vi "Simulation.vi"() -> ()   [LabVIEW 2012]
uses:
  <vilib>/Simulation/Scripting/Companion Diagram/SimConfigNode/SimParams.ctl
  <vilib>/Simulation/Scripting/Companion Diagram/SimConfigNode/_simSolvers.ctl
  <vilib>/Simulation/Implementation/Shared/SIMSCR Execution Mode.ctl
  <vilib>/Simulation/Param Hierarchy/Typedefs/SIMPH Param Control Actions.ctl
  <vilib>/Simulation/Implementation/Shared/NILVSim_ParamChanged.vi
  <vilib>/Simulation/ContinuousLinear/Implementation/NILVSim Transfer Function.llb/SIM Transfer Function Distributor (SISO).vi
  <vilib>/Simulation/DiscreteLinear/Implementation/NILVSim Discrete ZOH.llb/SIM Discrete ZOH (scalar).vi
  <vilib>/Simulation/Nonlinear/Implementation/NILVSim Relay.llb/SIM Relay (scalar).vi
  <vilib>/Simulation/ContinuousLinear/Implementation/NILVSim Transfer Function.llb/SIM Transfer Function Collector (SISO).vi
  <vilib>/Simulation/SignalDisplay/Implementation/NILVSim Time Waveform.llb/SIM Time Waveform (scalar).vi
  <vilib>/Simulation/Implementation/Shared/NILVSim_Manager.vi
  <vilib>/Simulation/Implementation/Shared/NILVSim_FinalizeModel.vi
  <vilib>/Simulation/Implementation/Shared/SIM Unbundle Sim Info.vi
  <vilib>/Utility/error.llb/Clear Errors.vi
  <vilib>/Simulation/Implementation/Shared/NILVSim_GetModelError.vi
  <vilib>/Simulation/Implementation/Shared/SIM Bundle Sim Info.vi
  <vilib>/Simulation/Implementation/Shared/SIMSH Read Queue.vi
  <vilib>/Simulation/Implementation/Shared/NILVSim_Initialize.vi
  <vilib>/Simulation/Utility/Implementation/NILVSim Get Time and IsAcceptedStep.vi
  <vilib>/Simulation/Scripting/Companion Diagram/SimConfigNode/SimDog.xnode
  <vilib>/Simulation/Implementation/XNodeFramework/SimXNode/SimX.xnode
  <vilib>/Simulation/ContinuousLinear/Implementation/NILVSim Transfer Function.llb/SIM Transfer Function (SISO).vi
  <vilib>/Simulation/Implementation/Shared/NI_SIM_Implementation.lvlib
panel:
  in  "sample  time":dbl
  in  "Lower Limit":dbl
  in  "Upper Limit":dbl
  in  "Off Voltage":dbl
  in  "Suply Voltage":dbl
  out "Output":dbl(slide) scale=0.0..5.0
  out "Controlled Variable (Plant output)":waveform(dbl)(graph)={"t0"=timestamp(9343.2 s since 1904-01-01), "dt"=1.0, "Y"=[0.2633720690985406]}
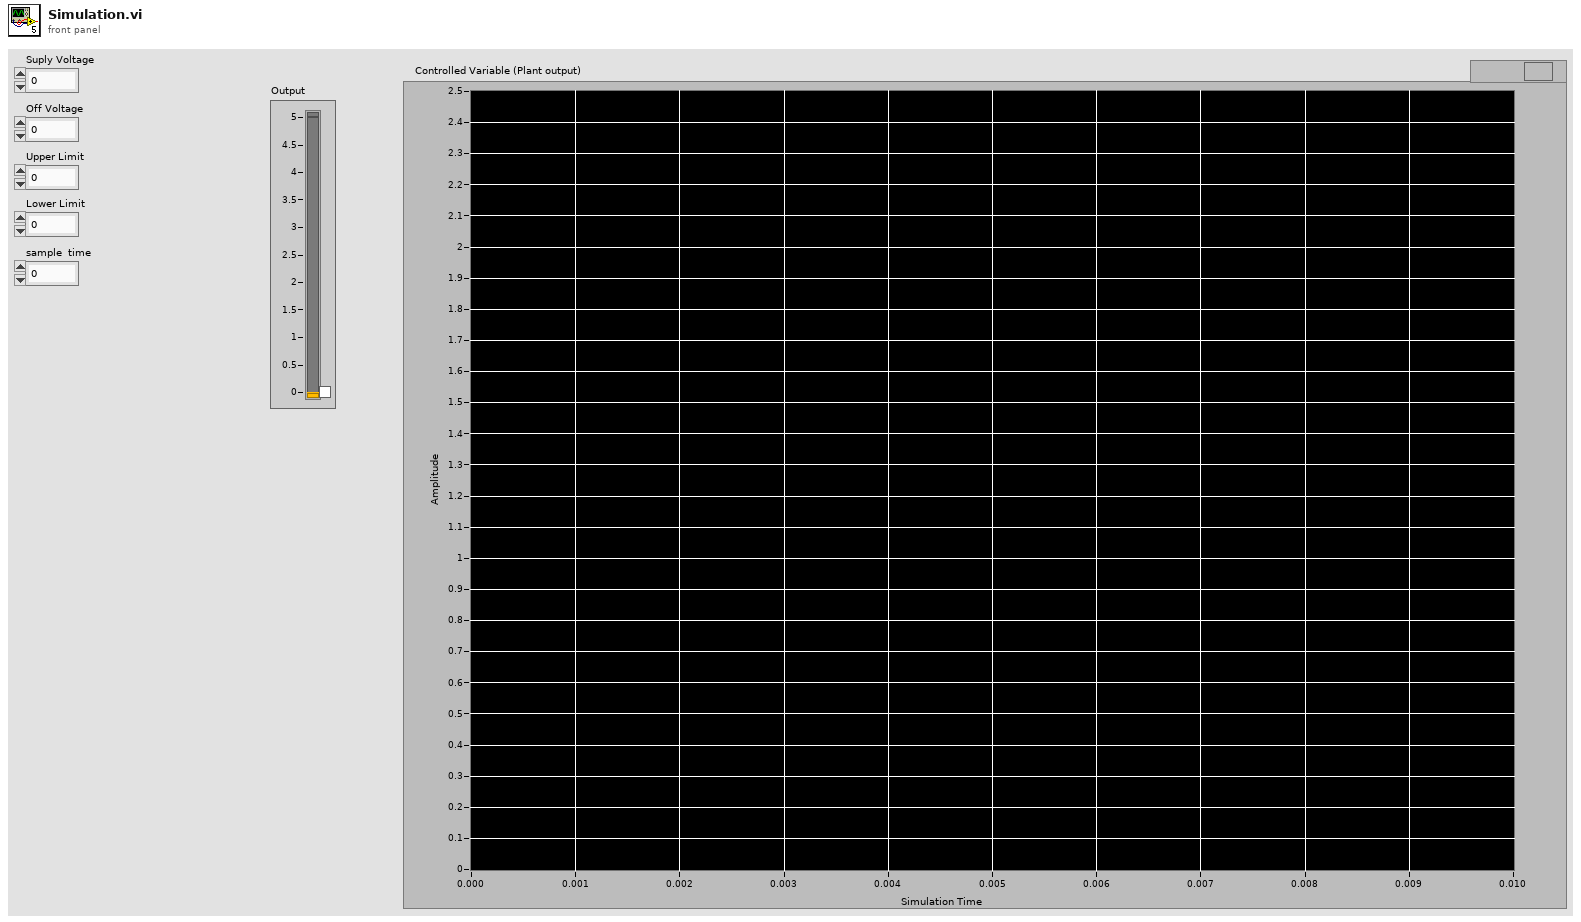
[diagram p1: front panel]
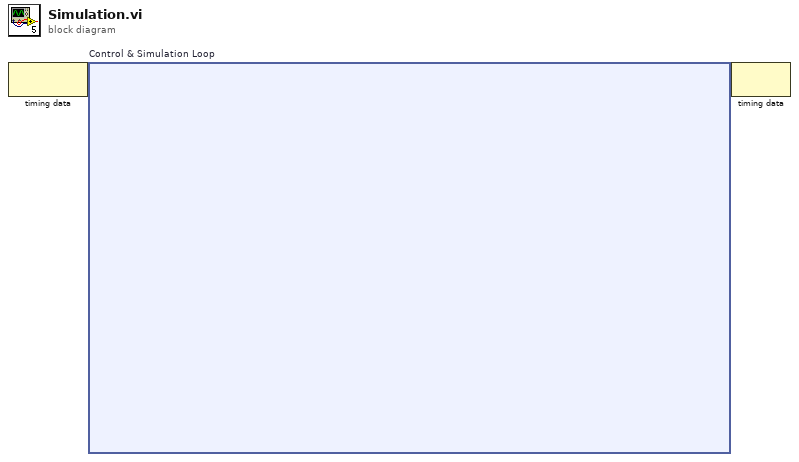
[diagram p0: block diagram]
diagram:
  n1 = node-c288() -> (w2:variant)  [unwired: 1 in]
  n2 = node-c254 "Control & Simulation Loop"(w2) -> (w1:variant)
  n3 = node-c288(w1) -> ()  [unwired: 1 out]
